vi "Limelight Set Camera Mode.vi"(11 "Camera Mode":enum16{"Vision Processor", "Driver Camera"}(ring)=enum."Driver Camera") -> (0 "error out":errorcluster)   [LabVIEW 2019]
uses:
  <vilib>/Rock Robotics/Network Tables/NT Write Number.vi
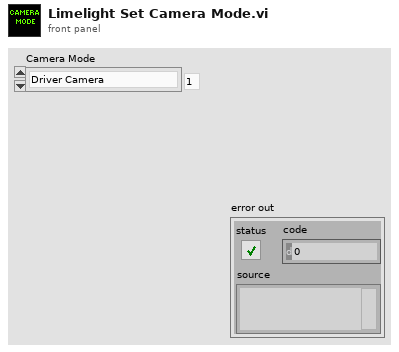
[diagram p1: front panel]
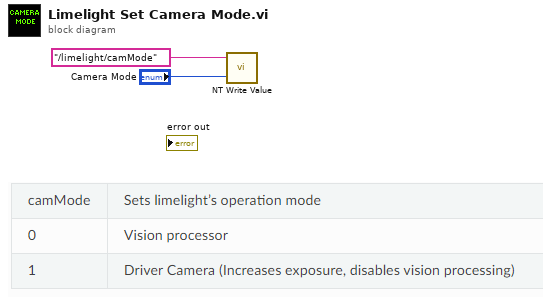
[diagram p0: block diagram]
diagram:
  n1 = call-poly <vilib>:"NT Write Value.vi"("Numeric"="Camera Mode", "Name"="/limelight/camMode") -> ()  [unwired: 9 in, 1 out]
